vi "Try Match Response.vi"(7 "Rcvd Event Regd":refnum<notifier>, 8 "error in":errorcluster, 10 "SDO Transfer":refnum<class "SDO Transfer.lvclass">, 11 "SDO Manager":refnum<class "SDO Manager.lvclass">) -> (0 "error out":errorcluster, 2 "SDO Result":T1={"Success"=FALSE, "SDO abort code"={"Null"=TRUE, "Value"=84082688}, "Data"={"Null"=TRUE, "Data"=[]}} {"SDO abort code"."Value" items=["Toggle bit not allowed"=84082688, "SDO protocol timed out"=84148224, "Client/server command specifier not valid or unknown"=84148225, "Invalid block size (block mode only)"=84148226, "Invalid sequence number (block mode only)"=84148227, "CRC error (block mode only)"=84148228, "Out of memory"=84148229, "Attempt to read a write only object"=100728833, "Attempt to write a read only object"=100728834, "Object does not exist in the object dictionary"=100794368, "Object cannot be mapped to the PDO"=100925505, "The number and length of the objects to be mapped would exceed PDO length"=100925506, "General parameter incompatibility reason"=100925507, "General internal incompatibility in the device"=100925511, "Access failed due to an hardware error"=101056512, "Data type does not match, length of service parameter does not match"=101122064, "Data type does not match, length of service parameter too high"=101122066, "Data type does not match, length of service parameter too low"=101122067, "Sub-index does not exist"=101253137, "Invalid value for parameter (download only)"=101253168, "Value of parameter written too high (download only)"=101253169, "Value of parameter written too low (download only)"=101253170, "Maximum value is less than minimum value"=101253174, "Resource not available: SDO connection"=101318691, "General error"=134217728, "Data cannot be transferred or stored to the application"=134217760, "Data cannot be transferred or stored to the application because of local control"=134217761, "Data cannot be transferred or stored to the application because of the present device stable"=134217762, "Object dictionary dynamic generation fails or no object dictionary is present (e.g. object dictionary is generated from file and generation fails because of an file error)"=134217763, "No data available"=134217764]; "Data"."Data" format="%02x"})   [LabVIEW 2020, in "CANopen.lvlib" / "SDO Manager.lvlib" / "SDO Manager.lvclass"]
uses:
  SDO Manager.lvclass
  SDO Transfer/SDO Transfer.lvclass
  D:/git/CANopen-LabVIEW/source/Response Matcher/IResponse/IMatch Response.lvclass
  SDO Manager.lvclass/SDO Manager.ctl
  SDO Transfer/SDO Transfer.lvclass/SDO Transfer.ctl
  HAL/Source/Interfaces/ICAN CC Frame/ICAN CC Frame.lvclass
  HAL/Source/Interfaces/ICommunicate/ICommunicate.lvclass
  Response Matcher/IResponse/IMatch Response.lvclass
  Logging/Log Level.vi
  Logging/CANopen Logging.lvlib
  SDO Transfer/SDO abort code.ctl
  Typedefs/SDO Result.ctl
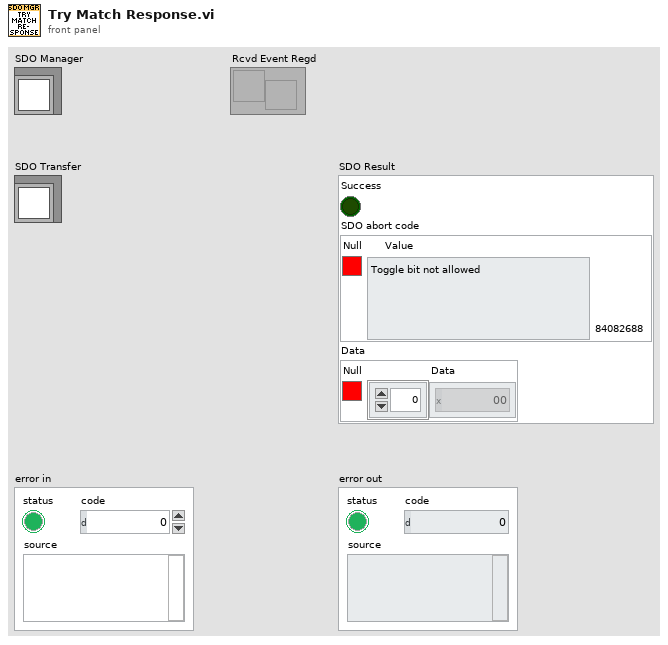
[diagram p1: front panel]
types:
  T1 = typedef "CANopen.lvlib/SDO Manager.lvlib/SDO Transfer.lvclass/SDO Result.ctl" = cluster{"Success":bool, "SDO abort code":cluster{"Null":bool, "Value":T2}, "Data":cluster{"Null":bool, "Data":u8[]}}
  T2 = typedef "CANopen.lvlib/SDO Manager.lvlib/SDO Transfer.lvclass/SDO abort code.ctl" = u32
  T3 = enum16{"Error", "Warn", "Info", "Debug", "Trace"}
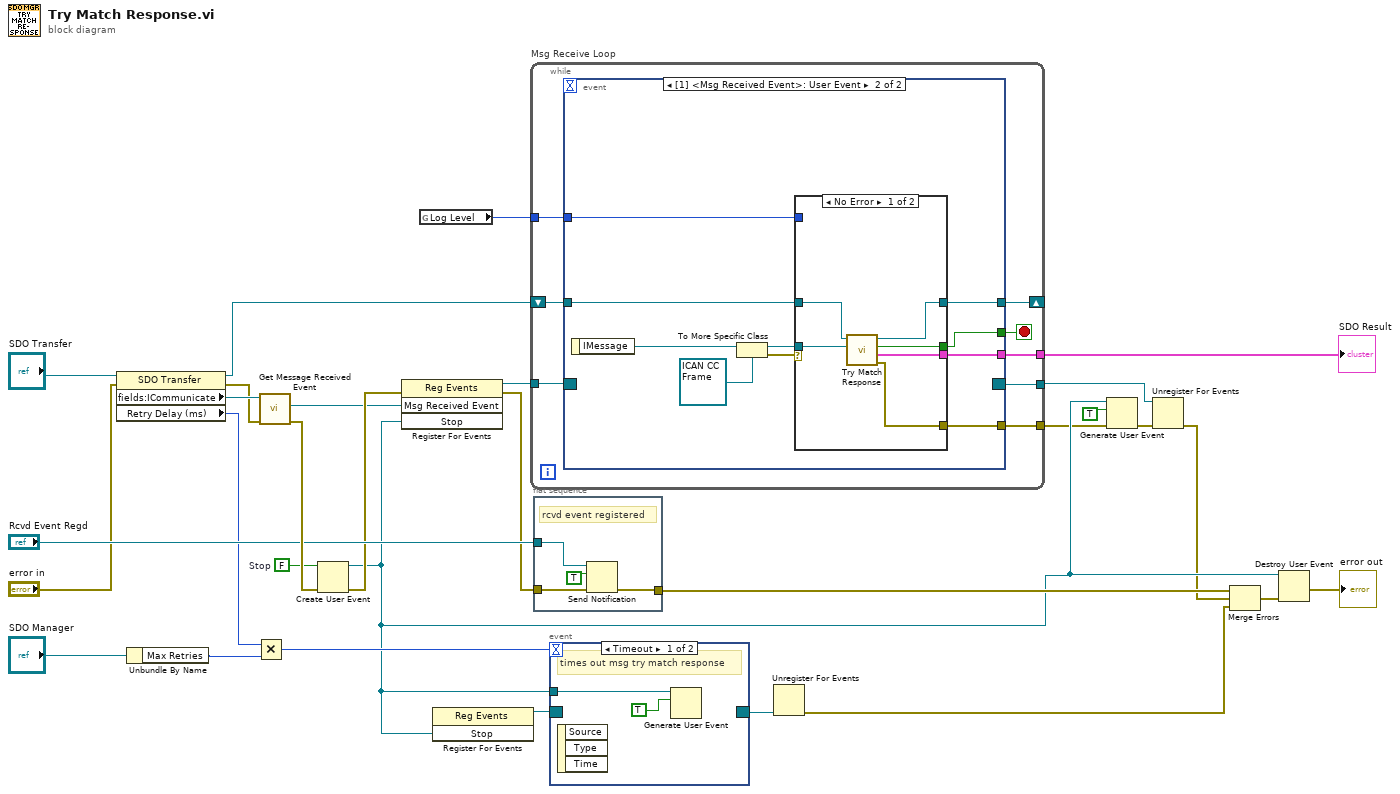
[diagram p0: block diagram]
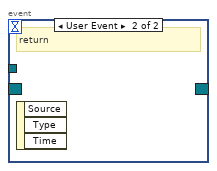
[diagram p2: hidden frame]
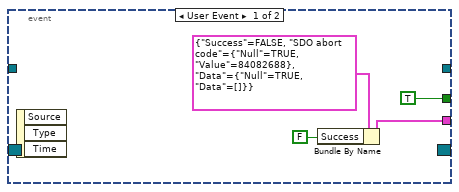
[diagram p3: hidden frame]
diagram:
  w22 = FALSE  # Stop
  n1 = property class="SDO Transfer"(reference="SDO Transfer", error in="error in") -> (reference out=w3:refnum<class "SDO Transfer.lvclass">, error out=w1:errorcluster, "fields:ICommunicate"=w18:refnum<class "ICommunicate.lvclass">, "Retry Delay (ms)"=w17:i32)
  n2 = Unbundle By Name("SDO Manager") -> ("Max Retries"=w19:u8)
  n3 = Multiply(x=w17, y=w19) -> (x*y=w15:i32)
  n4 = call-dynamic "Get Message Received Event.vi"("error in"=w1, "ICommunicate in"=w18) -> ("error out"=w30:errorcluster, "Msg Received Event"=w16:refnum<user-event>)  [unwired: 7 in, 1 out]
  n5 = Create User Event(user event datatype=w22, error in=w30) -> (user event=w8:refnum<user-event>, error out=w21:errorcluster)
  n6 = register-events(error in=w21, w16, w8) -> (reference out=w23:refnum<event-registration>, error out=w20:errorcluster)  [unwired: 1 in]
  n7 = global read "Log Level.vi" "Log Level"() -> (w24:T3)
  n8 = register-events(w8) -> (reference out=w14:refnum<event-registration>)  [unwired: 2 in, 1 out]
  n9 = while "Msg Receive Loop" {
    tunnel: w23 -> [w37]
    tunnel: [w36] -> w5
    tunnel: w24 -> [w35]
    shift-right: [w33] -> _
    shift-left: w3 -> [w34]
    tunnel: [w32] -> w26
    tunnel: [w31] -> w4
    stop <- w38 stop-if-true
    n10 = event shown="[1] <Msg Received Event>: User Event" {
      selector: w37 -> [_ _]
      dyn-events: [_ _] -> w36
      timeout: _ -> [_ _]
      tunnel: [TRUE w45] -> w38
      tunnel: w35 -> [_ w51]
      tunnel: w34 -> [_ w47]
      tunnel: [_ w46] -> w33
      tunnel: [w40 w44] -> w32
      tunnel: [_ w43] -> w31
      event User Event {
        n11 = event-data() -> ()  [unwired: 1 in, 3 out]
        n12 = Bundle By Name(cluster=T1 {"Success"=FALSE, "SDO abort code"={"Null"=TRUE, "Value"=84082688}, "Data"={"Null"=TRUE, "Data"=[]}} ("SDO Result"), "Success"=FALSE) -> (w40:T1)
      }
      event User Event {
        n13 = event-data() -> ("IMessage"=w52:refnum<class "IMessage.lvclass">)  [unwired: 1 in]
        n14 = To More Specific Class(target class=refnum<class "ICAN CC Frame.lvclass"> refnum ("ICAN CC Frame"), reference=w52) -> (specific class reference=w50:refnum<class "ICAN CC Frame.lvclass">, error out=w48:errorcluster)  [unwired: 1 in]
        n15 = case shown="No Error" w48 {
          tunnel: w47 -> [w58 w59]
          tunnel: w50 -> [w57 _]
          tunnel: w51 -> [_ _]
          tunnel: [w56 w59] -> w46
          tunnel: [w53 _] -> w45
          tunnel: [w55 _] -> w44
          tunnel: [w54 _] -> w43
          frame No Error {
            n16 = call-dynamic "Try Match Response.vi"("ICAN CC Frame"=w57, "SDO Transfer in"=w58) -> ("error out"=w54:errorcluster, "SDO Result"=w55:T1, "Match"=w53:bool, "IResponse out"=w56:refnum<class "IMatch Response.lvclass">)  [unwired: 6 in]
          }
          frame Error {
          }
        }
      }
    }
  }
  "SDO Result" <- w26
  n17 = flat-sequence {
    tunnel: w20 -> [w61]
    tunnel: "Rcvd Event Regd" -> [w63]
    tunnel: [w60] -> w11
    frame #0 {
      # "rcvd event registered"
      n18 = Send Notification(notification=TRUE, notifier=w63, error in (no error)=w61) -> (error out=w60:errorcluster)  [unwired: 1 out]
    }
  }
  n19 = event shown="[0] Timeout" {
    selector: w14 -> [_ _]
    dyn-events: [_ _] -> w13
    timeout: w15 -> [_ _]
    tunnel: w8 -> [w65 _]
    event Timeout {
      # "times out msg try match response"
      n20 = event-data() -> ()  [unwired: 1 in, 3 out]
      n21 = Generate User Event(user event=w65, event data cluster=TRUE) -> ()  [unwired: 2 in, 2 out]
    }
    event User Event {
      # "return"
      n22 = event-data() -> ()  [unwired: 1 in, 3 out]
    }
  }
  n23 = Unregister For Events(event registration refnum=w13) -> (error out=w10:errorcluster)  [unwired: 1 in]
  n24 = Generate User Event(user event=w8, event data cluster=TRUE ("event data"), error in=w4) -> (error out=w9:errorcluster)  [unwired: 1 in, 1 out]
  n25 = Unregister For Events(event registration refnum=w5, error in=w9) -> (error out=w6:errorcluster)
  n26 = Merge Errors(w11, w6, w10) -> (w12:errorcluster)
  n27 = Destroy User Event(user event=w8, error in=w12) -> (error out=→"error out":errorcluster)
